vi "Set Waveform Label.vi"(8 "error in (no error)":errorcluster, 9 "Label":string, 10 "Analog Channels":T1, 11 "MSOX6004 in":refnum<class "MSOX6004.lvclass">) -> (0 "error out":errorcluster, 3 "MSOX6004 out":refnum<class "MSOX6004.lvclass">)   [LabVIEW 2018, in "MSOX6004.lvlib" / "MSOX6004.lvclass"]
doc: "This Override is used to label channel waveforms."
uses:
  MSOX6004.lvclass
  PPLs/Oscilloscope/Parent/Oscilloscope.lvlibp/Custom Controls/Analog Channels.ctl
  MSOX6004.lvclass/MSOX6004.ctl
  <instrlib>/Keysight InfiniiVision/Keysight InfiniiVision.lvlib
  PPLs/Oscilloscope/Parent/Oscilloscope.lvlibp
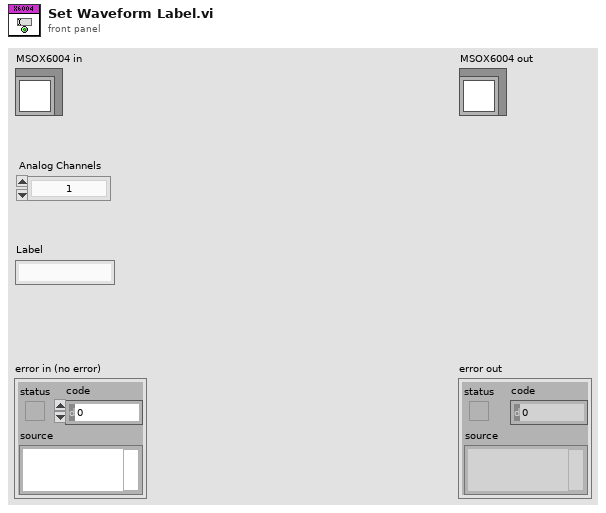
[diagram p1: front panel]
types:
  T1 = typedef "Oscilloscope.lvlibp/Analog Channels.ctl" = enum16{"1", "2", "3", "4", "5", "6", "7", "8", "9", "10", "11", "12", "13", "14", "15", "16"}
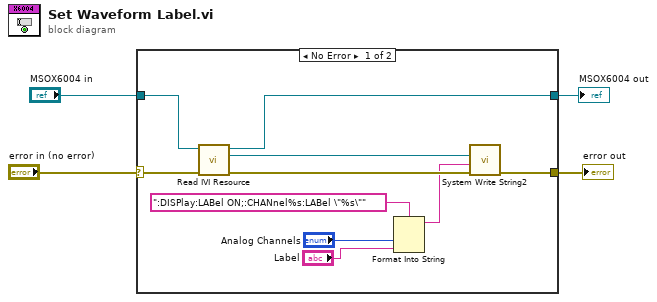
[diagram p0: block diagram]
diagram:
  n1 = case shown="No Error" "error in (no error)" {
    selector: "error in (no error)" -> [w13 w16]
    tunnel: [w5 w16] -> w3
    tunnel: [w9 w15] -> w2
    tunnel: "MSOX6004 in" -> [w12 w15]
    frame No Error {
      n2 = call "Read IVI Resource.vi"("error in (no error)"=w13, "MSOX6004 in"=w12) -> ("error out"=w8:errorcluster, "IVI Resource"=w7:refnum<k15>, "MSOX6004 out"=w9:refnum<class "MSOX6004.lvclass">)  [unwired: 7 in]
      n3 = Format Into String(format string=":DISPlay:LABel ON;:CHANnel%s:LABel \"%s\"", "Analog Channels", "Label") -> (resulting string=w6:string)  [unwired: 2 in, 1 out]
      n4 = call <instrlib>:"System Write String2.vi"("error in (no error)"=w8, "Data"=w6, "instrument handle"=w7) -> ("error out"=w5:errorcluster)  [unwired: 7 in, 1 out]
    }
    frame Error {
    }
  }
  "error out" <- w3
  "MSOX6004 out" <- w2
